vi "Configure Analog Alarm Parameters 1.vi"(0 "VISA resource name":refnum<visa-resource-name>, 1 "Unit Address (1)":u8=1, 2 "Alarm Number (1)":u16=1 min=1 max=8, 5 "Threshold (0)":u16=1 max=10000, 7 "Alarm Hysteresis (0)":u16 max=10000, 9 "Latching Mode (0: No Latch)":u16(ring)=1 items=["No Latch", "Automatic Latching", "Manual Latching", "Event Latching"], 11 "error in (no error)":errorcluster, 12 "Priority (1: Low Priority)":u8(ring)=1 items=["Low Priority"=1, "Medium Priority"=2, "High Priority"=3]) -> (4 "VISA resource name out":refnum<visa-resource-name>, 15 "error out":errorcluster)   [LabVIEW 2014, in "Eurotherm 35xx Series.lvlib"]
doc: "This VI Configure parameters of selected analog alarm (part 1)."
uses:
  <instrlib>/Eurotherm 35xx Series/Eurotherm 35xx Series.lvlib
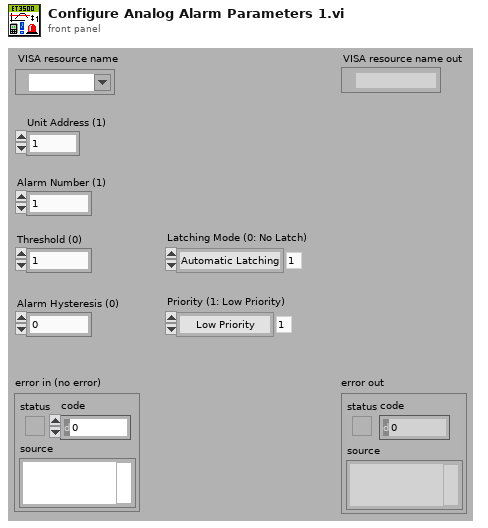
[diagram p1: front panel]
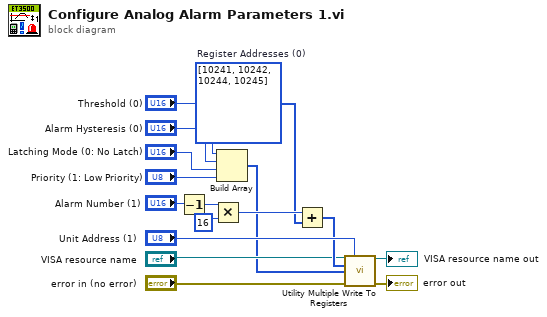
[diagram p0: block diagram]
diagram:
  w2 = u16[] [10241, 10242, 10244, 10245]  # Register Addresses (0)
  n1 = Decrement(x="Alarm Number (1)") -> (x-1=w15:u16)
  n2 = Multiply(x=w15, y=u16 16) -> (x*y=w5:u16)
  n3 = Build Array("Threshold (0)", "Alarm Hysteresis (0)", "Latching Mode (0: No Latch)", "Priority (1: Low Priority)") -> (w1:u16[])
  n4 = Add(x=w5, y=w2) -> (x+y=w6:u16[])
  n5 = call <instrlib>:"Utility Multiple Write To Registers.vi"("VISA resource name"="VISA resource name", "Unit Address (1)"="Unit Address (1)", "Registers Addresses (0)"=w6, "Data (0)"=w1, "error in (no error)"="error in (no error)") -> ("VISA resource name out"=→"VISA resource name out":refnum<visa-resource-name>, "error out"=→"error out":errorcluster)  [unwired: 9 in]
